vi "Configure Data Marker [DM] Core.vi"(6 "Destination Terminal (None)":string(combo) caption="destination terminal (None)", 7 "Bit Position":i32 caption="bit position" format="%.0g", 8 "error in (no error)":errorcluster, 9 "Marker Name (\"\")":string caption="marker name (\"\")", 10 "Source Channel (\"\")":string="CHANNEL1" caption="source channel (\"CHANNEL1\")", 11 "CS++Fgen in":refnum<class "CS++Fgen.lvclass">) -> (0 "error out":errorcluster, 3 "CS++Fgen out":refnum<class "CS++Fgen.lvclass">)   [LabVIEW 2015, in "CS++Fgen.lvlib" / "CS++Fgen.lvclass"]
doc: "This VI configures the common data marker properties. These properties are the data marker source channel, bit position, and destination.\n \nNote:\n\n(1) This VI is part of the IviFgenDataMarker [DM] extension group."
uses:
  CS++Fgen.lvclass
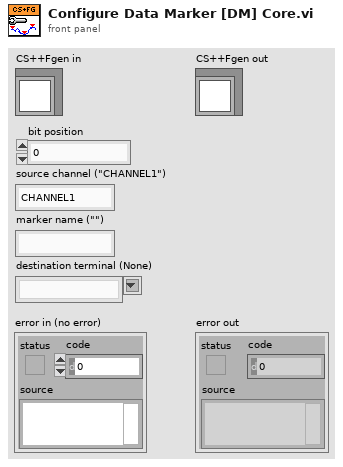
[diagram p1: front panel]
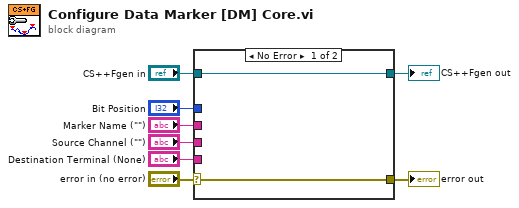
[diagram p0: block diagram]
diagram:
  n1 = case shown="No Error" "error in (no error)" {
    selector: "error in (no error)" -> [w9 w12]
    tunnel: [w9 w12] -> w7
    tunnel: [w10 w11] -> w5
    tunnel: "CS++Fgen in" -> [w10 w11]
    tunnel: "Bit Position" -> [_ _]
    tunnel: "Marker Name (\"\")" -> [_ _]
    tunnel: "Source Channel (\"\")" -> [_ _]
    tunnel: "Destination Terminal (None)" -> [_ _]
    frame No Error {
    }
    frame Error {
    }
  }
  "error out" <- w7
  "CS++Fgen out" <- w5
